vi "toggle and timing.vi"() -> ()   [LabVIEW 2020]
panel:
  out "Sweep Chart":dbl(graph)
  in  "timer on":bool
  in  "timer":dbl format="%.2f"
  in  "te":bool
  out "Clock":string="1:28:18 AM"
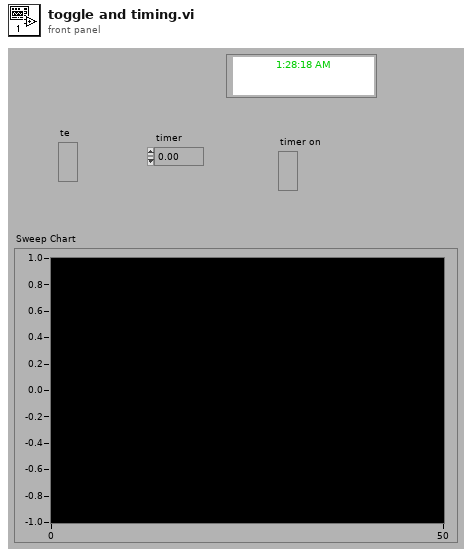
[diagram p1: front panel]
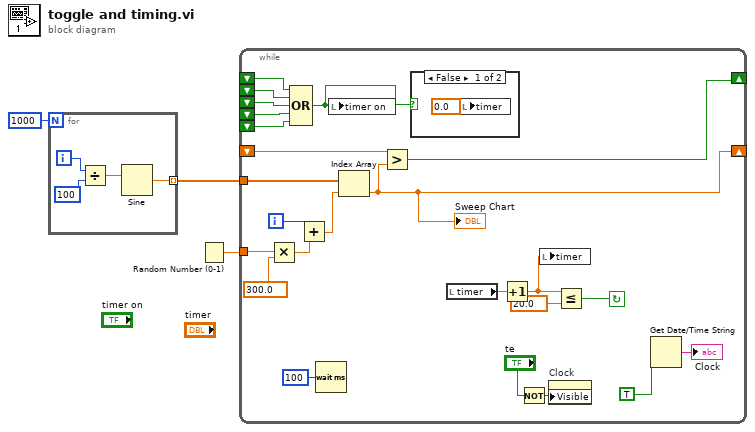
[diagram p0: block diagram]
diagram:
  n1 = for {
    N: 1000 -> [_]
    tunnel: [w4] -> w2 mode=indexing
    i -> [w7]
    n2 = Divide(x=w7, y=100) -> (x/y=w5:dbl)
    n3 = Sine(x=w5) -> (sin(x)=w4:dbl)
  }
  n4 = Random Number (0-1)() -> (number: 0 to 1=w1:dbl)
  n5 = while {
    shift-left: _ -> [w15]
    shift-left: _ -> [w16]
    shift-left: _ -> [w17]
    shift-left: _ -> [w18]
    shift-left: _ -> [w19]
    shift-right: [w20] -> _
    shift-left: _ -> [w21]
    shift-right: [w14] -> _
    tunnel: w1 -> [w26]
    tunnel: w2 -> [w23]
    i -> [w25]
    stop <- w8 continue-if-true
    n6 = Multiply(x=w26, y=300.0) -> (x*y=w24:dbl)
    n7 = Compound Arithmetic op=OR(w19, w18, w17, w16, w15) -> (w12:bool)
    n8 = Add(x=w25, y=w24) -> (x+y=w22:dbl)
    n9 = Wait (ms)(milliseconds to wait=u32 100) -> ()  [unwired: 1 out]
    n10 = local write "timer on"(w12) -> ()
    n11 = Index Array(array=w23, index=w22) -> (element=w14:dbl)
    "Sweep Chart" <- w14
    n12 = Greater?(x=w21, y=w14) -> (0:w20:bool)
    n13 = case shown="False" w12 {
      frame False {
        n14 = local write "timer"(0.0 ("timer")) -> ()
      }
      frame True {
      }
    }
    n15 = local read "timer"() -> (w11:dbl)
    n16 = Increment(x=w11) -> ()  [unwired: 1 out]
    n17 = Not(x="te") -> (.not. x?=w29:bool)
    n18 = local write "timer"(w11) -> ()
    n19 = property on="Clock" class="Str"("Visible"=w29) -> ()  [unwired: 2 in, 2 out]
    n20 = Less Or Equal?(x=w11, y=20.0) -> (x <= y?=w8:bool)
    n21 = Get Date/Time String(want seconds? (F)=TRUE) -> (time string=→"Clock":string)  [unwired: 2 in, 1 out]
  }
